vi "testSame.vi"() -> ()   [LabVIEW 2017, in "Assertion.Tests.lvlib" / "AssertNotEquals.lvlib"]
uses:
  AssertNotEquals.lvlib
  795a4de6-0cb0-48a6-807d-ef6fcaf9e1c4.vi
  Constraint/IsEqual/IsEqual.lvclass
  C:/Users/de200256/Code/logmanoriginal/lvunit/Constraint/Constraint/Constraint.lvclass
  Constraint/IsEqual/Create.vi
  Constraint/LogicalNot/LogicalNot.lvclass
  Constraint/UnaryOperator/UnaryOperator.lvclass
  Assertion/Assertion.lvlib
panel:
  out "error out":errorcluster
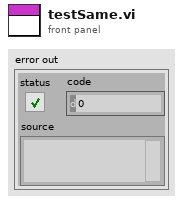
[diagram p1: front panel]
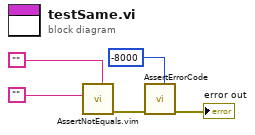
[diagram p0: block diagram]
diagram:
  n1 = call "AssertNotEquals.vim"("Expected"="", "Actual"="") -> ("error out"=w3:errorcluster)  [unwired: 9 in]
  n2 = call "AssertErrorCode.vi"("Expected"=-8000, "error in (no error)"=w3) -> ("error out"=→"error out":errorcluster)  [unwired: 9 in]
